vi "Build Parameter String.vi"(8 "error in (no error)":errorcluster, 10 "Parameters":T1[](array[typedef])) -> (0 "error out":errorcluster, 2 "Parameter String":string)   [LabVIEW 2011, in "i3-oauth.lvlib"]
doc: "Builds an OAuth parameter string from the supplied key-value pairs."
uses:
  i3-oauth.lvlib
  Controls/key-value-pairs.ctl
  i3-external-tools/i3-external-tools.lvlib
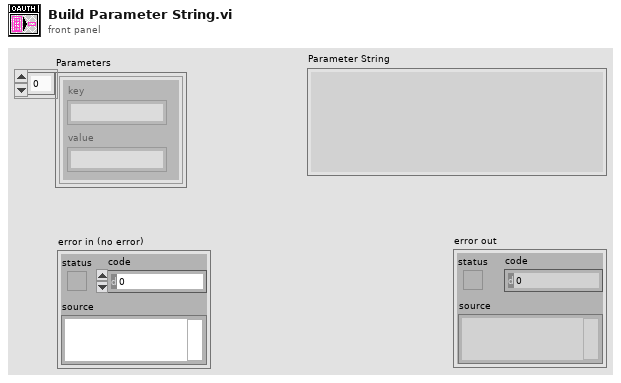
[diagram p1: front panel]
types:
  T1 = typedef "i3-oauth.lvlib/key-value-pairs.ctl" = cluster{"key":string, "value":string}
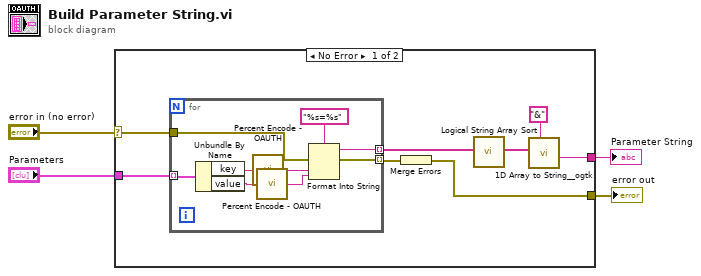
[diagram p0: block diagram]
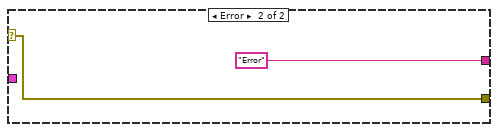
[diagram p2: hidden frame]
diagram:
  n1 = case shown="No Error" "error in (no error)" {
    selector: "error in (no error)" -> [w5 w23]
    tunnel: "Parameters" -> [w12 _]
    tunnel: [w7 "Error"] -> w3
    tunnel: [w6 w23] -> w2
    frame No Error {
      n2 = for {
        tunnel: w12 -> [w21] mode=indexing
        tunnel: [w17] -> w10 mode=indexing
        tunnel: w5 -> [w16]
        tunnel: [w15] -> w11 mode=indexing
        n3 = Unbundle By Name(w21) -> ("key"=w13:string, "value"=w20:string)
        n4 = call "Percent Encode - OAUTH.vi"("unescaped string in"=w13) -> ("escaped string out"=w14:string)
        n5 = call "Percent Encode - OAUTH.vi"("unescaped string in"=w20) -> ("escaped string out"=w18:string)
        n6 = Format Into String(format string="%s=%s", error in=w16, w14, w18) -> (resulting string=w17:string, error out=w15:errorcluster)  [unwired: 1 in]
      }
      n7 = Merge Errors(w11) -> (w6:errorcluster)
      n8 = call "Logical String Array Sort.vi"("Unsorted List"=w10) -> ("Sorted List"=w9:string[])  [unwired: 18 in]
      n9 = call <userlib>:"1D Array to String__ogtk.vi"("delimiter (Tab)"="&", "Array of Strings"=w9) -> ("delimited string"=w7:string)  [unwired: 9 in]
    }
    frame Error {
    }
  }
  "Parameter String" <- w3
  "error out" <- w2
